vi "MultislitCalc.vi"(5 "Slit Positions":T2, 7 "Star Positions":T3) -> (0 "test2":dbl, 1 "test1":dbl, 2 "Shifts":T1 {"Delta Theta" format="%#_3g"})   [LabVIEW 2015]
uses:
  SIcamera_Globals.vi
panel:
  out "Delta Theta":dbl format="%#_4g"
  out "Delta Theta 3":dbl format="%#_4g"
  out "Delta Theta 2":dbl format="%#_4g"
  out "Delta Theta 1":dbl format="%#_4g"
  in  "Y_0":i32=1465
  in  "X_0":i32=1568
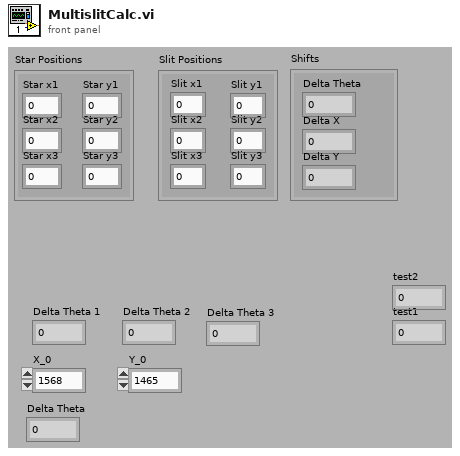
[diagram p1: front panel]
types:
  T1 = cluster{"Delta Theta":dbl, "Delta X":dbl, "Delta Y":dbl}
  T2 = cluster{"Slit x1":dbl, "Slit x2":dbl, "Slit x3":dbl, "Slit y2":dbl, "Slit y3":dbl, "Slit y1":dbl}
  T3 = cluster{"Star x1":dbl, "Star x2":dbl, "Star x3":dbl, "Star y2":dbl, "Star y3":dbl, "Star y1":dbl}
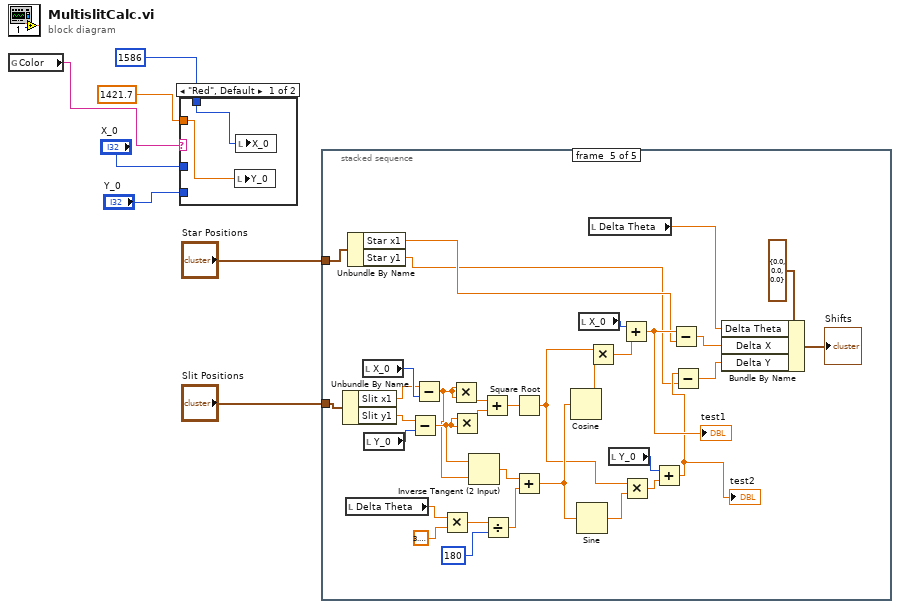
[diagram p0: block diagram]
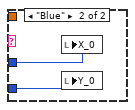
[diagram p2: hidden frame]
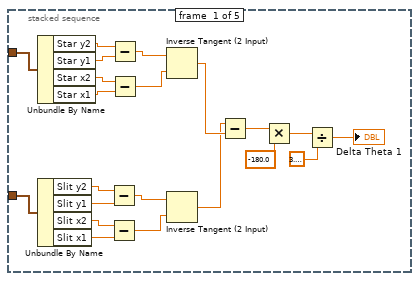
[diagram p3: hidden frame]
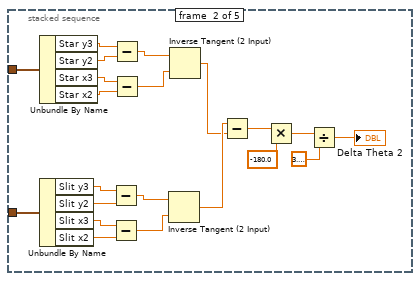
[diagram p4: hidden frame]
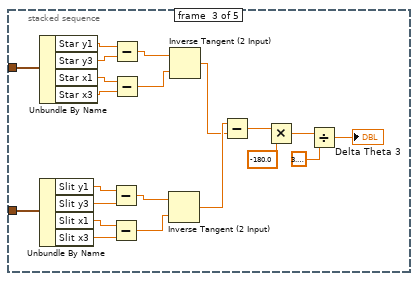
[diagram p5: hidden frame]
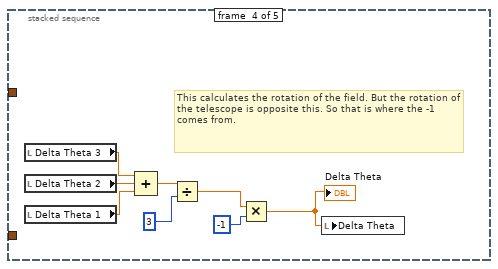
[diagram p6: hidden frame]
diagram:
  n1 = global read "SIcamera_Globals.vi" "Color"() -> (w1:string)
  n2 = case shown="\"Red\", Default" w1 {
    tunnel: "X_0" -> [_ w11]
    tunnel: "Y_0" -> [_ w10]
    tunnel: 1421.7 -> [w9 _]
    tunnel: 1586 -> [w8 _]
    frame "Red", Default {
      n3 = local write "Y_0"(w9) -> ()
      n4 = local write "X_0"(w8) -> ()
    }
    frame "Blue" {
      n5 = local write "X_0"(w11) -> ()
      n6 = local write "Y_0"(w10) -> ()
    }
  }
  n7 = stacked-sequence {
    tunnel: "Star Positions" -> [w32 w35 w56 _ w116]
    tunnel: "Slit Positions" -> [w31 w34 w55 _ w89]
    frame #0 {
      n8 = Unbundle By Name(w32) -> ("Star y2"=w28:dbl, "Star y1"=w27:dbl, "Star x2"=w30:dbl, "Star x1"=w29:dbl)
      n9 = Unbundle By Name(w31) -> ("Slit y2"=w26:dbl, "Slit y1"=w25:dbl, "Slit x2"=w24:dbl, "Slit x1"=w23:dbl)
      n10 = Subtract(x=w26, y=w25) -> (x-y=w14:dbl)
      n11 = Subtract(x=w24, y=w23) -> (x-y=w12:dbl)
      n12 = Subtract(x=w28, y=w27) -> (x-y=w15:dbl)
      n13 = Subtract(x=w30, y=w29) -> (x-y=w13:dbl)
      n14 = Inverse Tangent (2 Input)(1:w13, 2:w15) -> (0:w17:dbl)
      n15 = Inverse Tangent (2 Input)(1:w12, 2:w14) -> (0:w16:dbl)
      n16 = Subtract(x=w16, y=w17) -> (x-y=w21:dbl)
      n17 = Multiply(x=w21, y=-180.0) -> (x*y=w19:dbl)
      n18 = Divide(x=w19, y=3.141592653589793) -> (x/y=→"Delta Theta 1":dbl)
    }
    frame #1 {
      n19 = Unbundle By Name(w35) -> ("Star y3"=w49:dbl, "Star y2"=w48:dbl, "Star x3"=w51:dbl, "Star x2"=w50:dbl)
      n20 = Unbundle By Name(w34) -> ("Slit y3"=w45:dbl, "Slit y2"=w44:dbl, "Slit x3"=w43:dbl, "Slit x2"=w42:dbl)
      n21 = Subtract(x=w45, y=w44) -> (x-y=w47:dbl)
      n22 = Subtract(x=w43, y=w42) -> (x-y=w46:dbl)
      n23 = Subtract(x=w49, y=w48) -> (x-y=w53:dbl)
      n24 = Subtract(x=w51, y=w50) -> (x-y=w52:dbl)
      n25 = Inverse Tangent (2 Input)(1:w46, 2:w47) -> (0:w41:dbl)
      n26 = Inverse Tangent (2 Input)(1:w52, 2:w53) -> (0:w40:dbl)
      n27 = Subtract(x=w41, y=w40) -> (x-y=w38:dbl)
      n28 = Multiply(x=w38, y=-180.0) -> (x*y=w36:dbl)
      n29 = Divide(x=w36, y=3.141592653589793) -> (x/y=→"Delta Theta 2":dbl)
    }
    frame #2 {
      n30 = Unbundle By Name(w56) -> ("Star y1"=w70:dbl, "Star y3"=w69:dbl, "Star x1"=w72:dbl, "Star x3"=w71:dbl)
      n31 = Unbundle By Name(w55) -> ("Slit y1"=w66:dbl, "Slit y3"=w65:dbl, "Slit x1"=w64:dbl, "Slit x3"=w63:dbl)
      n32 = Subtract(x=w66, y=w65) -> (x-y=w68:dbl)
      n33 = Subtract(x=w64, y=w63) -> (x-y=w67:dbl)
      n34 = Subtract(x=w70, y=w69) -> (x-y=w74:dbl)
      n35 = Subtract(x=w72, y=w71) -> (x-y=w73:dbl)
      n36 = Inverse Tangent (2 Input)(1:w67, 2:w68) -> (0:w62:dbl)
      n37 = Inverse Tangent (2 Input)(1:w73, 2:w74) -> (0:w61:dbl)
      n38 = Subtract(x=w62, y=w61) -> (x-y=w59:dbl)
      n39 = Multiply(x=w59, y=-180.0) -> (x*y=w57:dbl)
      n40 = Divide(x=w57, y=3.141592653589793) -> (x/y=→"Delta Theta 3":dbl)
    }
    frame #3 {
      # "This calculates the rotation of the field. But the rotation of the telescope is opposite this. So that is where the -1 comes from."
      n41 = local read "Delta Theta 3"() -> (w82:dbl)
      n42 = local read "Delta Theta 2"() -> (w81:dbl)
      n43 = local read "Delta Theta 1"() -> (w80:dbl)
      n44 = Compound Arithmetic op=ADD(w82, w81, w80) -> (w79:dbl)
      n45 = Divide(x=w79, y=3) -> (x/y=w77:dbl)
      n46 = Multiply(x=w77, y=-1) -> (x*y=w75:dbl)
      "Delta Theta" <- w75
      n47 = local write "Delta Theta"(w75) -> ()
    }
    frame #4 {
      n48 = Unbundle By Name(w89) -> ("Slit x1"=w84:dbl, "Slit y1"=w83:dbl)
      n49 = local read "Delta Theta"() -> (w108:dbl)
      n50 = Unbundle By Name(w116) -> ("Star x1"=w86:dbl, "Star y1"=w85:dbl)
      n51 = local read "X_0"() -> (w114:i32)
      n52 = local read "Y_0"() -> (w115:i32)
      n53 = Subtract(x=w83, y=w115) -> (x-y=w110:dbl)
      n54 = Subtract(x=w84, y=w114) -> (x-y=w109:dbl)
      n55 = Multiply(x=w108, y=3.141592653589793) -> (x*y=w106:dbl)
      n56 = Multiply(x=w109, y=w109) -> (x*y=w113:dbl)
      n57 = Multiply(x=w110, y=w110) -> (x*y=w112:dbl)
      n58 = Inverse Tangent (2 Input)(1:w109, 2:w110) -> (0:w104:dbl)
      n59 = Add(x=w113, y=w112) -> (x+y=w111:dbl)
      n60 = Divide(x=w106, y=180) -> (x/y=w103:dbl)
      n61 = Square Root(x=w111) -> (sqrt(x)=w99:dbl)
      n62 = Add(x=w104, y=w103) -> (x+y=w101:dbl)
      n63 = Cosine(x=w101) -> (cos(x)=w102:dbl)
      n64 = Sine(x=w101) -> (sin(x)=w100:dbl)
      n65 = local read "X_0"() -> (w98:i32)
      n66 = Multiply(x=w99, y=w102) -> (x*y=w97:dbl)
      n67 = local read "Delta Theta"() -> (w90:dbl)
      n68 = local read "Y_0"() -> (w96:i32)
      n69 = Add(x=w98, y=w97) -> (x+y=w88:dbl)
      "test1" <- w88
      n70 = Multiply(x=w99, y=w100) -> (x*y=w95:dbl)
      n71 = Add(x=w96, y=w95) -> (x+y=w87:dbl)
      "test2" <- w87
      n72 = Subtract(x=w88, y=w86) -> (x-y=w92:dbl)
      n73 = Subtract(x=w87, y=w85) -> (x-y=w91:dbl)
      n74 = Bundle By Name(cluster=T1 {"Delta Theta"=0.0, "Delta X"=0.0, "Delta Y"=0.0} ("Shifts"), "Delta Theta"=w90, "Delta X"=w92, "Delta Y"=w91) -> (→"Shifts":T1)
    }
  }
